vi "main.vi"(11 "librarian_sm.lvclass":refnum<class "librarian.lvclass">) -> ()   [LabVIEW 2020, in "librarian.lvclass"]
uses:
  librarian.lvclass
  typedefs/library--map.ctl
  typedefs/lib_map_value--cluster.ctl
  typedefs/book_state--enum.ctl
  shared/message--cluster.ctl
  shared/request--enum.ctl
  librarian.lvclass/librarian.ctl
  shared/_JKI_lib_State_Machine.llb/Select State(s)_err__jki_lib_state_machine.vi
panel:
  out "error out":errorcluster[](array[cluster])
  out "log":string
  in  "Exit":bool
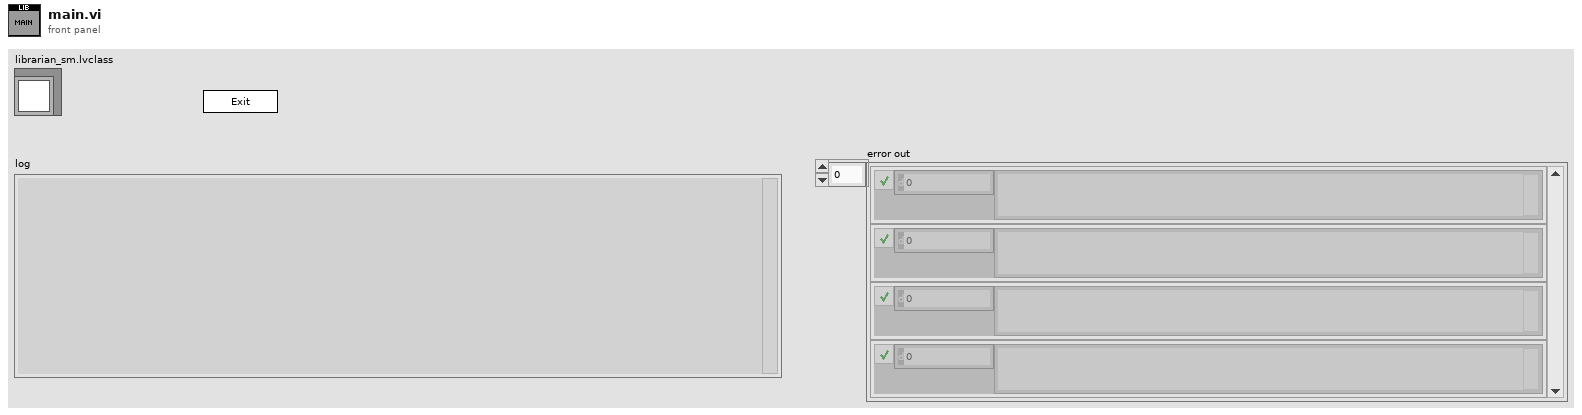
[diagram p1: front panel]
types:
  T1 = enum32{"Invalid", "Standard", "Closed", "Hidden", "Minimized", "Maximized"}
  T2 = enum32{"invalid app kind", "Development System", "Run Time System", "Student Edition", "Embedded LabVIEW", "Evaluation", "Custom"}
  T3 = typedef "librarian.lvclass/book_state--enum.ctl" = enum16{"CHECKEDIN", "CHECKEDOUT", "DAMAGED"}
  T4 = typedef "message--cluster.ctl" = cluster{"header":string, "cmd":T5, "title":string, "book":string}
  T5 = typedef "request--enum.ctl" = enum16{"CHECKIN", "CHECKOUT"}
  T6 = typedef "librarian.lvclass/lib_map_value--cluster.ctl" = cluster{"book state":T3, "text":string, "hash":string}
  T7 = typedef "librarian.lvclass/library--map.ctl" = map{string, T6}
  T8 = cluster{"Core":cluster{"Current VI Reference":refnum<vi>, "Close Panel on Exit?":bool}, "librarian_sm.lvclass":refnum<class "librarian.lvclass">, "TO":i32, "library map":T7, "listener ref":refnum<k5>, "client ref":refnum<k5>, "message":T4, "client map":map{string, cluster{"banned":bool, "title":string}}, "start time":u32}
  T9 = map{string, cluster{"banned":bool, "title":string}}
  T10 = cluster{"Current VI Reference":refnum<vi>, "Close Panel on Exit?":bool}
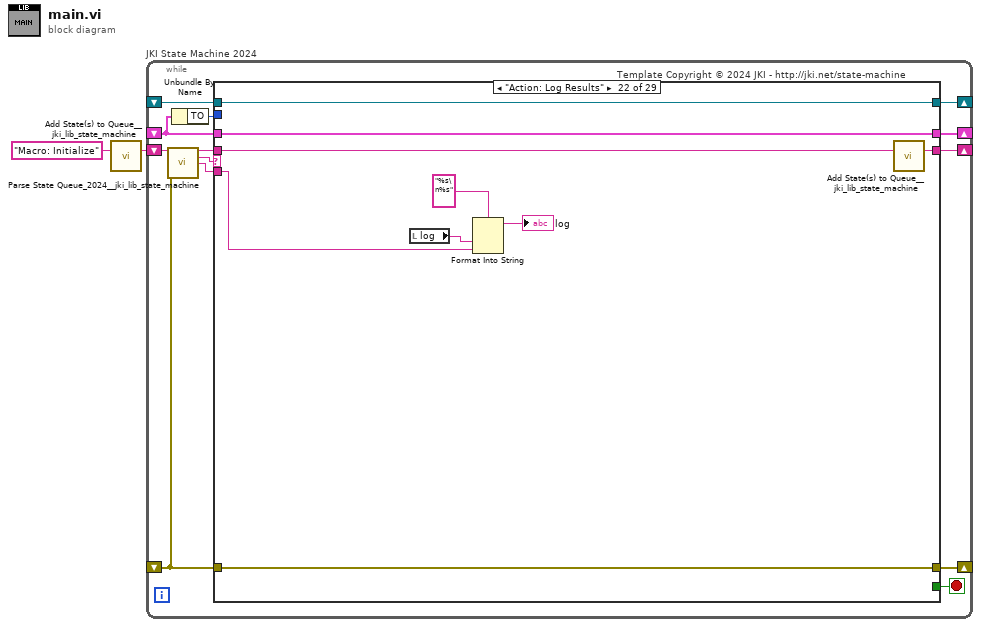
[diagram p0: block diagram]
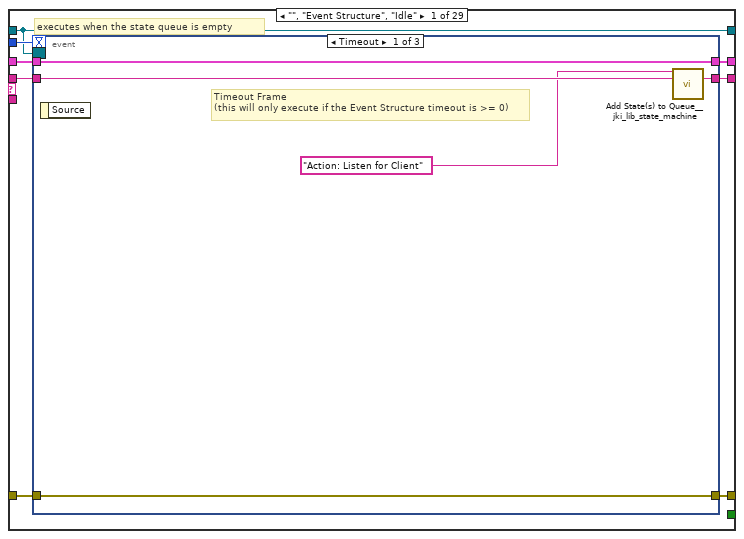
[diagram p2: hidden frame]
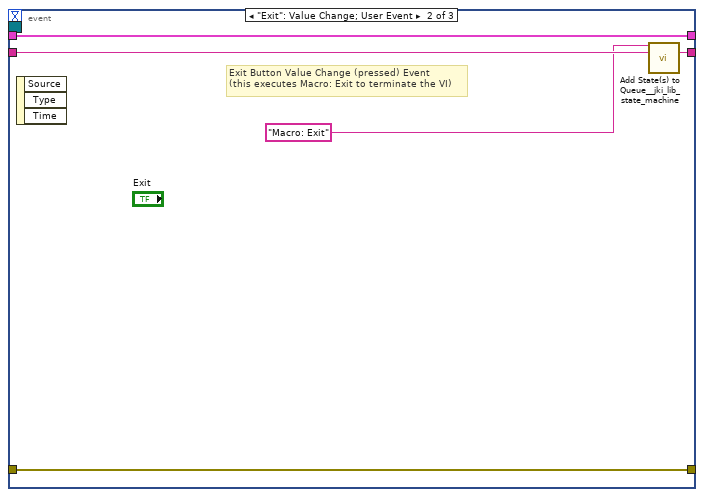
[diagram p3: hidden frame]
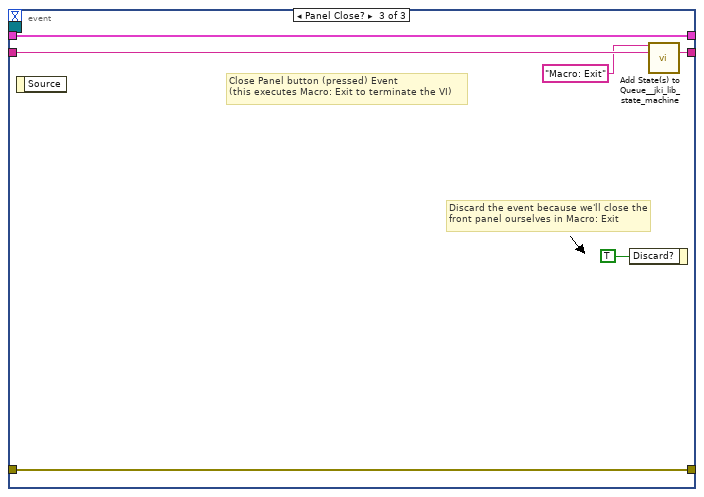
[diagram p4: hidden frame]
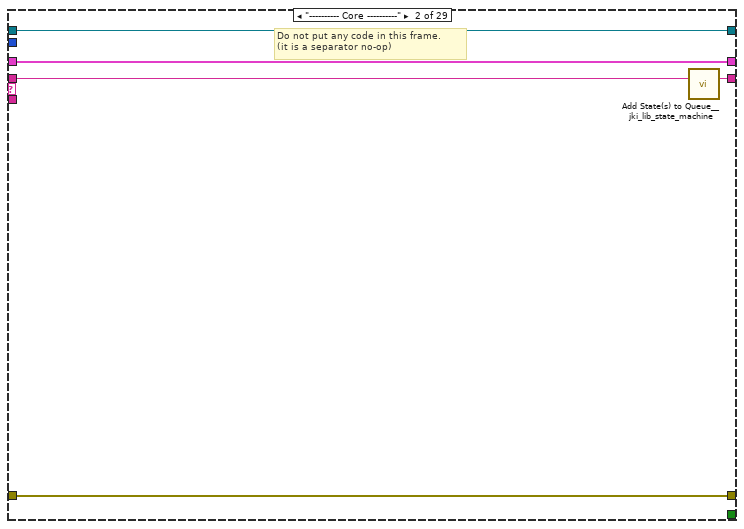
[diagram p5: hidden frame]
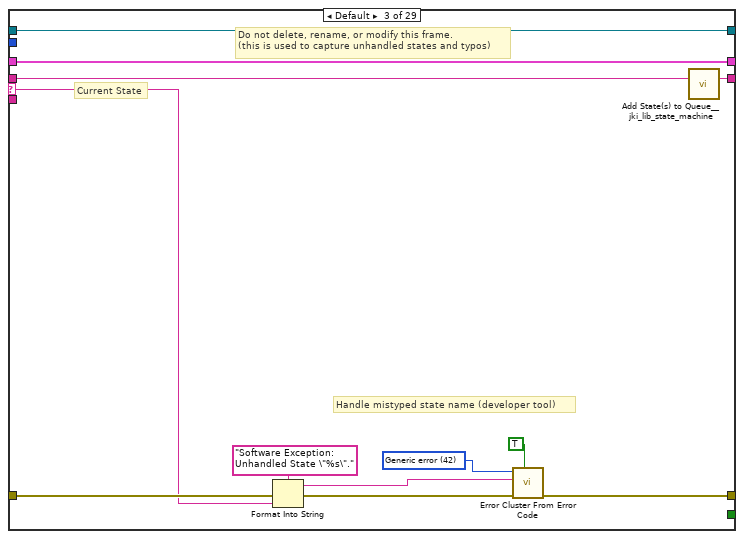
[diagram p6: hidden frame]
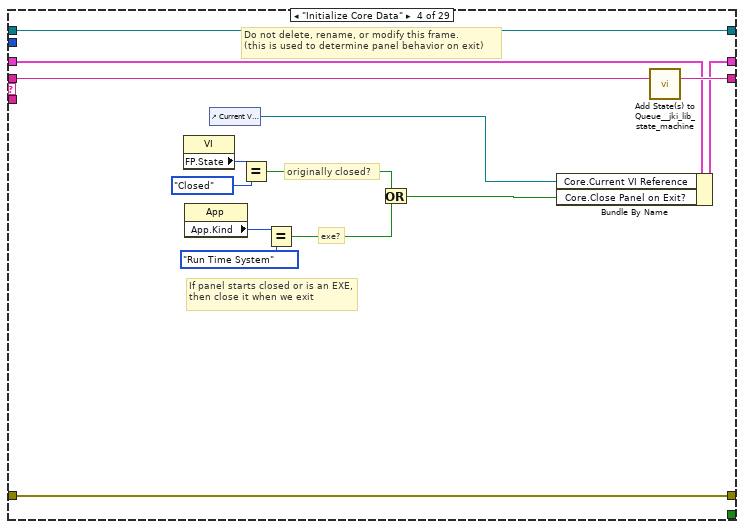
[diagram p7: hidden frame]
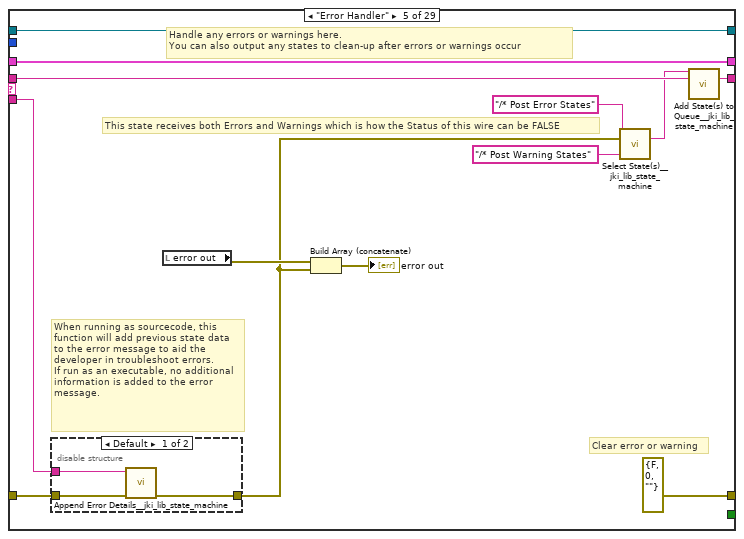
[diagram p8: hidden frame]
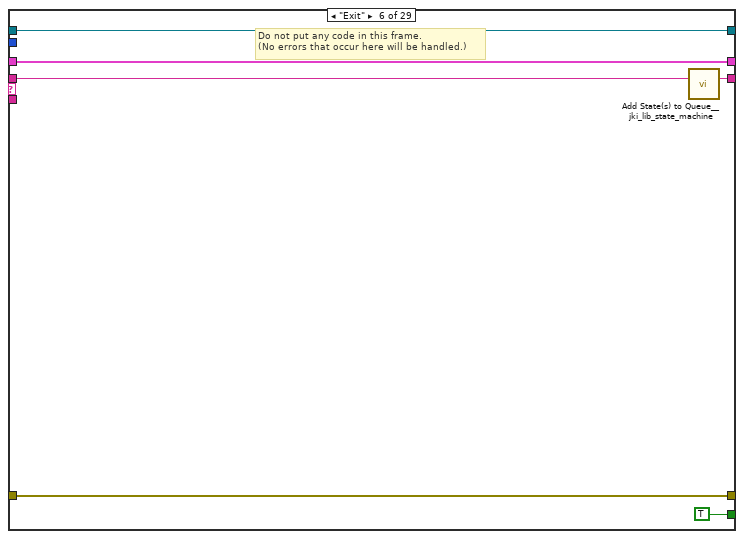
[diagram p10: hidden frame]
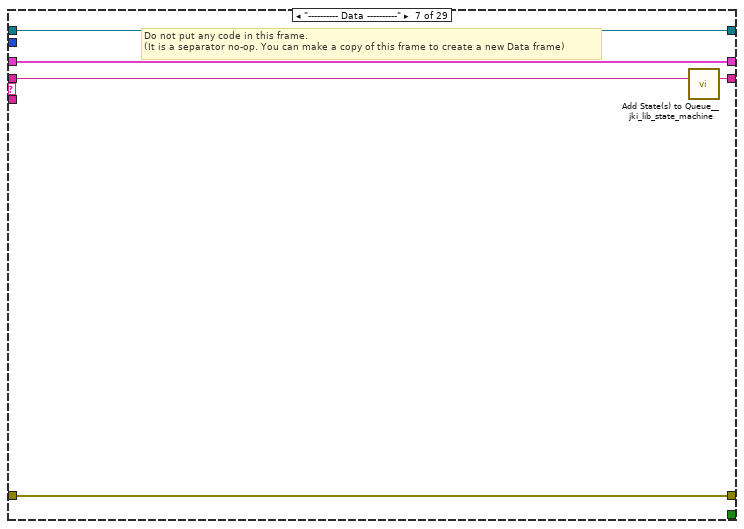
[diagram p11: hidden frame]
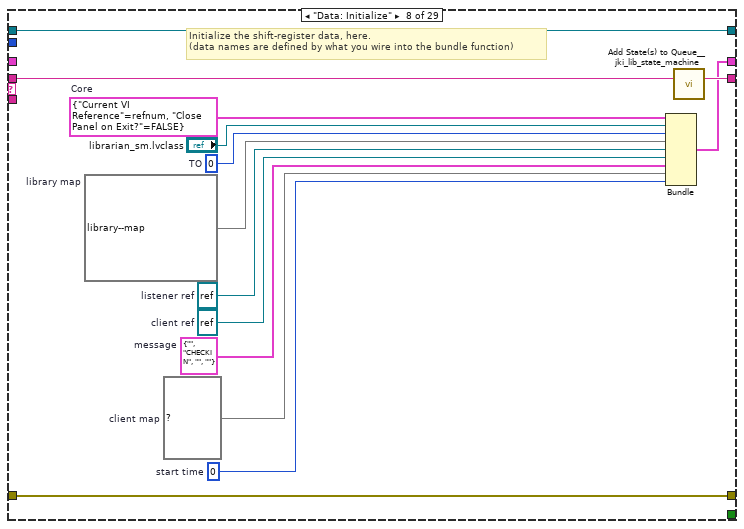
[diagram p12: hidden frame]
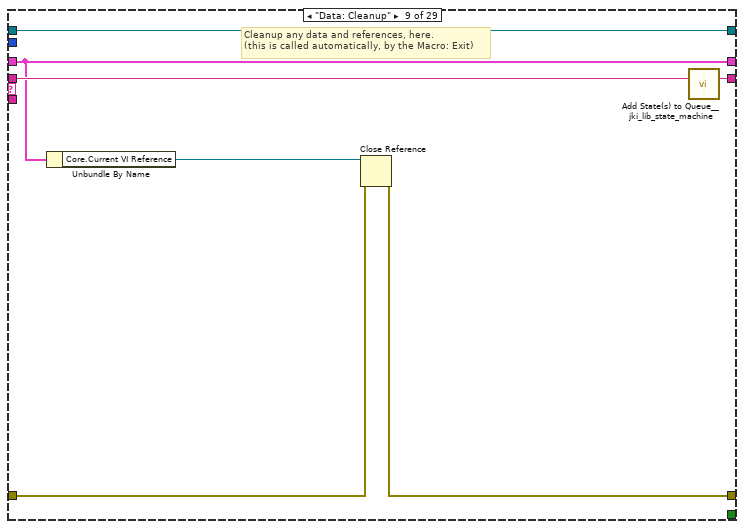
[diagram p13: hidden frame]
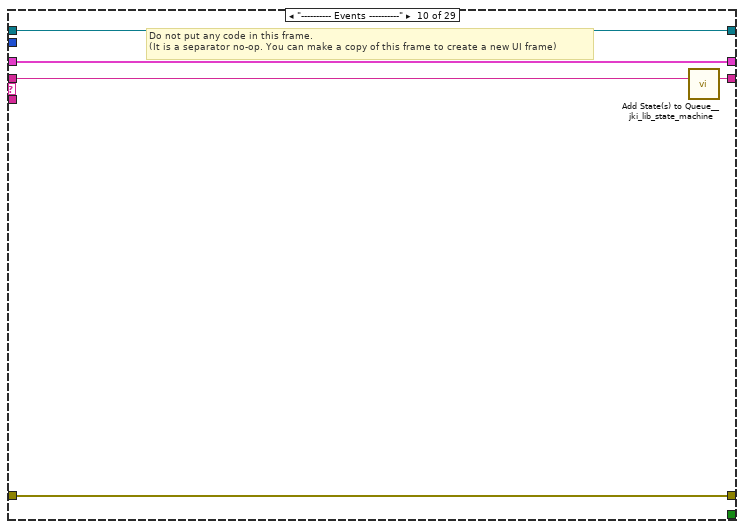
[diagram p14: hidden frame]
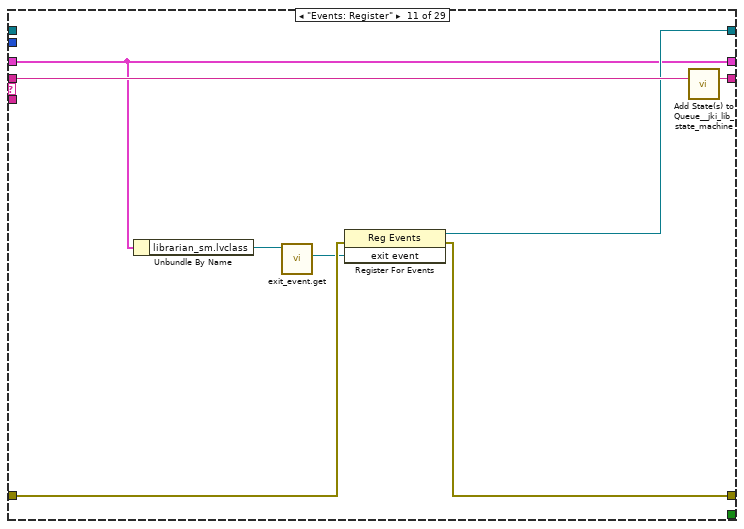
[diagram p15: hidden frame]
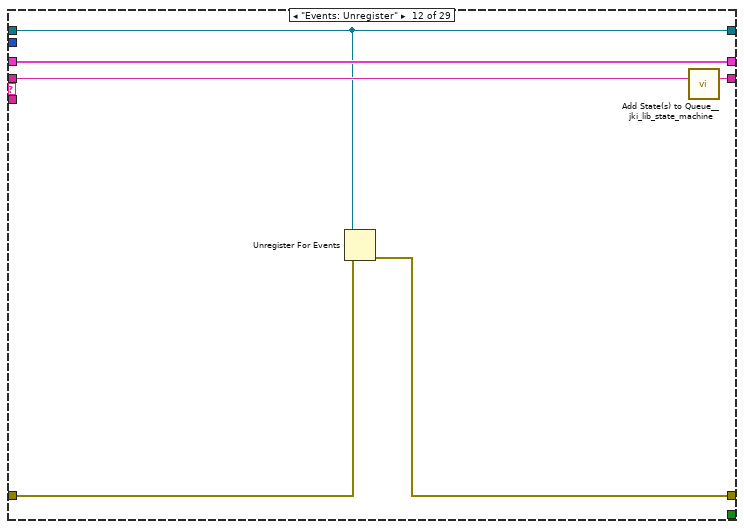
[diagram p16: hidden frame]
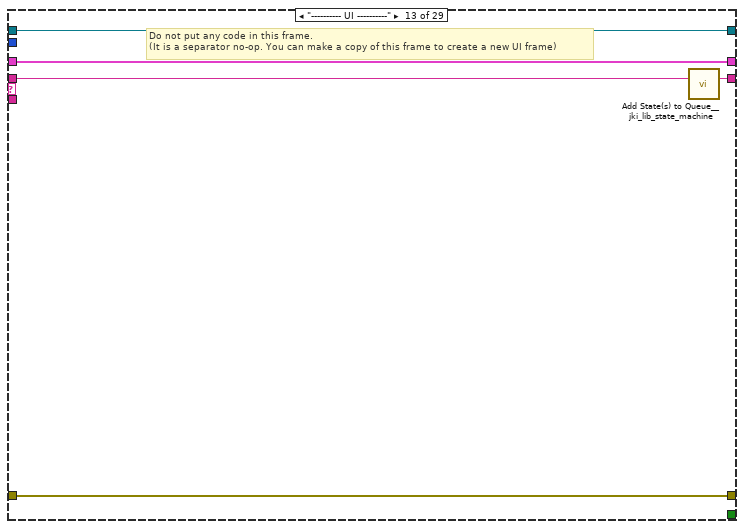
[diagram p17: hidden frame]
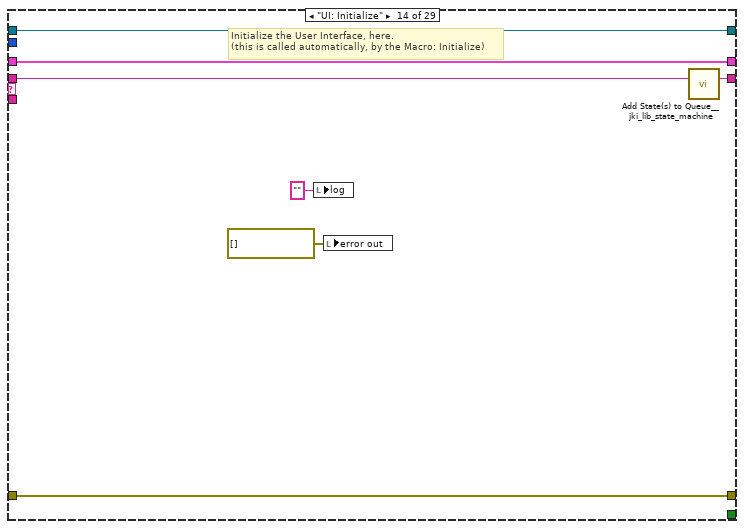
[diagram p18: hidden frame]
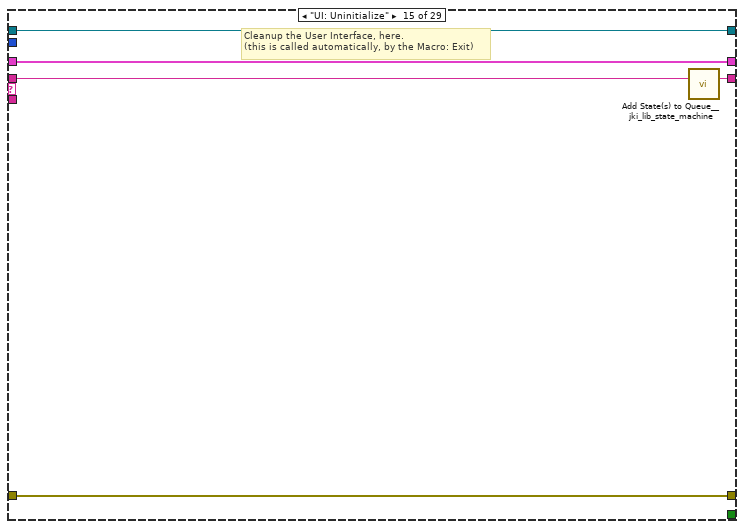
[diagram p19: hidden frame]
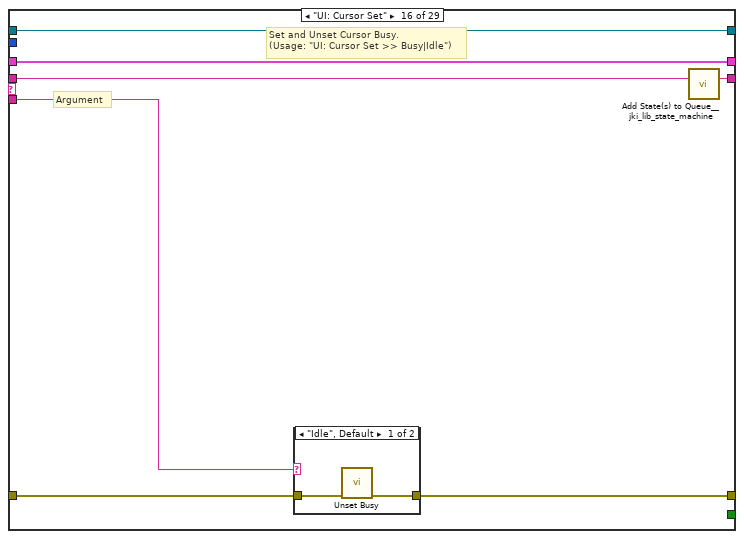
[diagram p20: hidden frame]
diagram:
  n1 = call "Add State(s) to Queue__jki_lib_state_machine.vi"("State(s) in (\"\")"="Macro: Initialize") -> ("States Out"=w2:string)  [unwired: 14 in]
  n2 = while "JKI State Machine 2024" {
    shift-right: [w8] -> _
    shift-left: _ -> [w4]
    shift-right: [w11] -> _
    shift-left: _ -> [w7]
    shift-right: [w10] -> _
    shift-left: w2 -> [w12]
    shift-right: [w6] -> _
    shift-left: _ -> [w5]
    stop <- w9 stop-if-true
    # "Template Copyright © 2024 JKI - http://jki.net/state-machine"
    n3 = call "Parse State Queue_2024__jki_lib_state_machine.vi"("State Queue"=w12, "Error In (no error)"=w7) -> ("Remaining States"=w14:string, "Current State"=w15:string, "Arguments"=w13:string)  [unwired: 11 in]
    n4 = Unbundle By Name(w4) -> ("TO"=w3:i32)
    n5 = case shown="\"Action: Log Results\"" w15 {
      selector: w15 -> [_ _ w46 _ _ _ _ _ _ _ _ _ _ _ _ _ _ _ _ _ _ _ _ _ _ _ _ _ _]
      tunnel: w14 -> [w23 w44 w50 w70 w83 w93 w98 w112 w119 w124 w132 w138 w143 w150 w155 w162 w174 w244 w250 w260 w265 w274 w295 w316 w363 w381 w406 w422 w434]
      tunnel: w13 -> [_ _ _ _ w78 _ _ _ _ _ _ _ _ _ _ w157 w168 _ _ _ _ w267 w283 _ _ _ _ _ _]
      tunnel: w4 -> [w21 w41 w48 w63 w80 w91 w95 _ w114 w121 w127 w136 w140 w148 w153 w160 w170 w241 w247 w258 w262 w271 w289 w307 w347 w370 w398 w419 w431]
      tunnel: [w20 w42 w52 w67 errorcluster {"status"=FALSE, "code"=0, "source"=""} ("error out") w90 w96 w109 w115 w122 w128 w133 w141 w147 w152 w158 w171 w242 w248 w255 w263 w272 w286 w314 w349 w367 w400 w416 w423] -> w11
      tunnel: w7 -> [w17 w42 w51 w67 w79 w90 w96 w109 w116 w122 w129 w134 w141 w147 w152 w159 w172 w242 w248 w255 w263 w272 w281 w314 w353 w375 w402 w417 w430]
      tunnel: [w22 w43 w49 w69 w82 w92 w97 w111 w118 w123 w131 w137 w142 w149 w154 w161 w173 w243 w249 w259 w264 w273 w294 w315 w362 w380 w405 w421 w433] -> w10
      tunnel: [_ _ _ _ _ TRUE _ _ _ _ _ _ _ _ _ _ _ _ _ _ _ _ _ _ _ _ _ _ _] -> w9
      tunnel: [w19 w41 w48 w68 w80 w91 w95 w110 w114 w121 w127 w136 w140 w148 w153 w160 w170 w241 w247 w258 w262 w271 w287 w305 w345 w369 w397 w419 w426] -> w8
      tunnel: w3 -> [w18 _ _ _ _ _ _ _ _ _ _ _ _ _ _ _ _ _ _ _ _ _ _ _ _ _ _ _ _]
      tunnel: [w16 w40 w45 w57 w74 w88 w94 w107 w113 w120 w130 w135 w139 w146 w151 w156 w167 w240 w245 w251 w261 w270 w293 w313 w361 w379 w404 w420 w432] -> w6
      tunnel: w5 -> [w16 w40 w45 w57 w74 w88 w94 w107 w113 w120 _ w135 w139 w146 w151 w156 w167 w240 w245 w251 w261 w270 w293 w313 w361 w379 w404 w420 w432]
      frame "", "Event Structure", "Idle" {
        # "executes when the state queue is empty"
        n6 = event shown="[0] Timeout" {
          selector: w16 -> [_ _ _]
          dyn-events: _ -> [_ _ _]
          timeout: w18 -> [_ _ _]
          tunnel: w23 -> [w28 w33 w39]
          tunnel: [w27 w32 w38] -> w22
          tunnel: w21 -> [w25 w30 w36]
          tunnel: [w26 w31 w37] -> w20
          tunnel: w17 -> [w26 w31 w37]
          tunnel: [w25 w30 w36] -> w19
          event Timeout {
            # "Timeout Frame\n(this will only execute if the Event Structure timeout is >= 0)"
            n7 = event-data() -> ()  [unwired: 1 in, 1 out]
            n8 = call "Add State(s) to Queue__jki_lib_state_machine.vi"("State(s) in Front (\"\")"="Action: Listen for Client" ("State"), "State(s) in (\"\")"=w28) -> ("States Out"=w27:string)  [unwired: 13 in]
          }
          event "Exit": Value Change; User Event {
            # "Exit Button Value Change (pressed) Event\n(this executes Macro: Exit to terminate the VI)"
            n9 = event-data() -> ()  [unwired: 1 in, 3 out]
            n10 = call "Add State(s) to Queue__jki_lib_state_machine.vi"("State(s) in Front (\"\")"="Macro: Exit", "State(s) in (\"\")"=w33) -> ("States Out"=w32:string)  [unwired: 13 in]
          }
          event Panel Close? {
            # "Discard the event because we'll close the front panel ourselves in Macro: Exit"
            # "Close Panel button (pressed) Event\n(this executes Macro: Exit to terminate the VI)"
            n11 = event-data() -> ()  [unwired: 1 in, 1 out]
            n12 = event-data("Discard?"=TRUE) -> ()  [unwired: 1 in, 1 out]
            n13 = call "Add State(s) to Queue__jki_lib_state_machine.vi"("State(s) in Front (\"\")"="Macro: Exit", "State(s) in (\"\")"=w39) -> ("States Out"=w38:string)  [unwired: 13 in]
          }
        }
      }
      frame "---------- Core ----------" {
        # "Do not put any code in this frame.\n(it is a separator no-op)"
        n14 = call "Add State(s) to Queue__jki_lib_state_machine.vi"("State(s) in (\"\")"=w44) -> ("States Out"=w43:string)  [unwired: 14 in]
      }
      frame Default {
        w55 = 42 items=["No error", "Argument error", "Memory is full", "Out of zone", "End of file", "File already open", "Generic file I/O error", "File not found", "File permission error", "Disk is full", "Duplicate path", "Too many files open", "System feature not enabled", "Resource file not found", "Cannot add resource", "Resource not found", "Image not found", "Image memory error", "Pen does not exist", "Config type invalid", "Config token not found", "Config parse error", "Config memory error", "Bad external code format", "Bad external code offset", "External code not present", "Null window", "Destroy window error", "Null menu", "Print aborted", "Bad print record", "Print driver error", "Windows error during printing", "Memory error during printing", "Print dialog error", "Generic print error", "Invalid device refnum", "Device not found", "Device parameter error", "Device unit error", "Cannot open device", "Device call aborted", "Generic error", "Cancelled by user", "Object ID too low", "Object ID too high", "Object not in heap", "Unknown heap", "Unknown object (invalid DefProc)", "Unknown object (DefProc not in table)", "Message out of range", "Invalid (null) method", "Unknown message", "Manager call not supported", "Bad address", "Network operation in progress", "Network operation timed out", "Connection is busy", "Network attribute not supported", "Network error", "Address in use", "System out of memory", "Connection aborted", "Connection refused", "Not connected", "Already connected", "Connection closed", "Initialization error (interapplication manager)", "Bad occurrence", "Wait on unbound occurrence handler", "Occurrence queue overflow", "Datalog type conflict", "Unused", "Unrecognized type (interapplication manager)", "Memory corrupt", "Failed to make temporary DLL", "Old CIN version", "Drag socket not found", "Failed to load drop-object", "Failed to register OLE object", "Failed to release OLE object", "Format specifier type mismatch", "Unknown format specifier", "Too few format specifiers", "Too many format specifiers", "Scan failed", "Newer CIN version", "Error converting to variant", "Runtime menu error", "Password tampered", "Variant attribute not found", "Incompatible variant data type", "Event data is not available", "Event Store is not present", "Occurrence is not found", "Event Queue is not created", "Event info is not available", "Refnum passed is NULL", "Error retrieving Class GUID", "Error retrieving CoClass GUID", "Error retrieving TypeLib GUID.", "Bad built application magic bytes.", "Specific driver is different from the specific driver associated with the Logical Name.", "There is no session opened to the class driver.", "Max Error", "MAX - Error with config objects", "MAX - Error loading configuration", "MAX - Group not supported"]
        # "Current State"
        # "Do not delete, rename, or modify this frame.\n(this is used to capture unhandled states and typos)"
        # "Handle mistyped state name (developer tool)"
        n15 = Format Into String(format string="Software Exception: Unhandled State \"%s\"." ("message"), error in=w51, w46) -> (resulting string=w54:string, error out=w53:errorcluster)  [unwired: 1 in]
        n16 = call <vilib>:"Error Cluster From Error Code.vi"("show call chain? (False)"=TRUE, "error in (no error)"=w53, "error message (\"\")"=w54, "error code (0)"=w55) -> ("error out"=w52:errorcluster)  [unwired: 5 in]
        n17 = call "Add State(s) to Queue__jki_lib_state_machine.vi"("State(s) in (\"\")"=w50) -> ("States Out"=w49:string)  [unwired: 14 in]
      }
      frame "Initialize Core Data" {
        # "Do not delete, rename, or modify this frame.\n(this is used to determine panel behavior on exit)"
        # "originally closed?"
        # "exe?"
        # "If panel starts closed or is an EXE, then close it when we exit"
        n18 = property class="VI"() -> ("FP.State"=w60:T1)  [unwired: 2 in, 2 out]
        n19 = property class="App"() -> ("App.Kind"=w66:T2)  [unwired: 2 in, 2 out]
        n20 = control-ref of="Current VI Reference"() -> (w61:refnum<vi>)
        n21 = Equal?(x=w60, y=T1."Closed" ("Front Panel Window:State")) -> (x = y?=w58:bool)
        n22 = Equal?(x=w66, y=T2."Run Time System" ("Application:Kind")) -> (x = y?=w64:bool)
        n23 = Or(x=w58, y=w64) -> (x .or. y?=w62:bool)
        n24 = Bundle By Name(cluster=w63, "Core.Current VI Reference"=w61, "Core.Close Panel on Exit?"=w62) -> (w68:T8)
        n25 = call "Add State(s) to Queue__jki_lib_state_machine.vi"("State(s) in (\"\")"=w70) -> ("States Out"=w69:string)  [unwired: 14 in]
      }
      frame "Error Handler" {
        # "When running as sourcecode, this function will add previous state data to the error message to aid the developer in troubleshoot errors.\nIf run as an executable, no additional information is added to the error message."
        # "This state receives both Errors and Warnings which is how the Status of this wire can be FALSE"
        # "Handle any errors or warnings here.\nYou can also output any states to clean-up after errors or warnings occur"
        # "Clear error or warning"
        n26 = disable-structure shown="Default" {
          disable-tunnel: w79 -> [w86 w87]
          disable-tunnel: w78 -> [w85 _]
          disable-tunnel: [w84 w87] -> w72
          frame condition #0 (active) {
            n27 = call "Append Error Details__jki_lib_state_machine.vi"("error in (no error)"=w86, "Previous State and Argument(s)"=w85) -> ("error out"=w84:errorcluster)  [unwired: 9 in]
          }
          frame condition #1 {
          }
        }
        n28 = local read "error out"() -> (w73:errorcluster[])
        n29 = Build Array (concatenate)(w73, w72) -> (→"error out":errorcluster[])
        n30 = call-poly "Select State(s)__jki_lib_state_machine.vi"("State(s) if True (\"\")"="/* Post Error States", "Select"=w72, "State(s) if False (\"\")"="/* Post Warning States") -> ("States Out"=w76:string)  [unwired: 12 in]
        n31 = call "Add State(s) to Queue__jki_lib_state_machine.vi"("State(s) in Front (\"\")"=w76, "State(s) in (\"\")"=w83) -> ("States Out"=w82:string)  [unwired: 13 in]
      }
      frame "Exit" {
        # "Do not put any code in this frame.\n(No errors that occur here will be handled.)"
        n32 = call "Add State(s) to Queue__jki_lib_state_machine.vi"("State(s) in (\"\")"=w93) -> ("States Out"=w92:string)  [unwired: 14 in]
      }
      frame "---------- Data ----------" {
        # "Do not put any code in this frame.\n(It is a separator no-op. You can make a copy of this frame to create a new Data frame)"
        n33 = call "Add State(s) to Queue__jki_lib_state_machine.vi"("State(s) in (\"\")"=w98) -> ("States Out"=w97:string)  [unwired: 14 in]
      }
      frame "Data: Initialize" {
        w99 = u32 0  # start time
        w100 = T9 {}  # client map
        w101 = T4 {"header"="", "cmd"=enum."CHECKIN", "title"="", "book"=""}  # message
        w102 = refnum<k5> refnum  # client ref
        w103 = refnum<k5> refnum  # listener ref
        w104 = T7 {}  # library map
        w105 = 0  # TO
        w108 = T10 {"Current VI Reference"=refnum, "Close Panel on Exit?"=FALSE}  # Core
        # "Initialize the shift-register data, here.\n(data names are defined by what you wire into the bundle function)"
        n34 = Bundle("Core"=w108, "librarian_sm.lvclass"="librarian_sm.lvclass", "TO"=w105, "library map"=w104, "listener ref"=w103, "client ref"=w102, "message"=w101, "client map"=w100, "start time"=w99) -> (w110:T8)  [unwired: 1 in]
        n35 = call "Add State(s) to Queue__jki_lib_state_machine.vi"("State(s) in (\"\")"=w112) -> ("States Out"=w111:string)  [unwired: 14 in]
      }
      frame "Data: Cleanup" {
        # "Cleanup any data and references, here.\n(this is called automatically, by the Macro: Exit)"
        n36 = Unbundle By Name(w114) -> ("Core.Current VI Reference"=w117:refnum<vi>)
        n37 = Close Reference(reference=w117, error in (no error)=w116) -> (error out=w115:errorcluster)
        n38 = call "Add State(s) to Queue__jki_lib_state_machine.vi"("State(s) in (\"\")"=w119) -> ("States Out"=w118:string)  [unwired: 14 in]
      }
      frame "---------- Events ----------" {
        # "Do not put any code in this frame.\n(It is a separator no-op. You can make a copy of this frame to create a new UI frame)"
        n39 = call "Add State(s) to Queue__jki_lib_state_machine.vi"("State(s) in (\"\")"=w124) -> ("States Out"=w123:string)  [unwired: 14 in]
      }
      frame "Events: Register" {
        n40 = Unbundle By Name(w127) -> ("librarian_sm.lvclass"=w126:refnum<class "librarian.lvclass">)
        n41 = call "exit_event.get.vi"("librarian_sm in"=w126) -> ("exit event"=w125:refnum<user-event>)  [unwired: 9 in, 1 out]
        n42 = register-events(error in=w129, w125) -> (reference out=w130:refnum<event-registration>, error out=w128:errorcluster)  [unwired: 1 in]
        n43 = call "Add State(s) to Queue__jki_lib_state_machine.vi"("State(s) in (\"\")"=w132) -> ("States Out"=w131:string)  [unwired: 14 in]
      }
      frame "Events: Unregister" {
        n44 = Unregister For Events(event registration refnum=w135, error in=w134) -> (error out=w133:errorcluster)
        n45 = call "Add State(s) to Queue__jki_lib_state_machine.vi"("State(s) in (\"\")"=w138) -> ("States Out"=w137:string)  [unwired: 14 in]
      }
      frame "---------- UI ----------" {
        # "Do not put any code in this frame.\n(It is a separator no-op. You can make a copy of this frame to create a new UI frame)"
        n46 = call "Add State(s) to Queue__jki_lib_state_machine.vi"("State(s) in (\"\")"=w143) -> ("States Out"=w142:string)  [unwired: 14 in]
      }
      frame "UI: Initialize" {
        # "Initialize the User Interface, here.\n(this is called automatically, by the Macro: Initialize)"
        n47 = local write "log"("" ("log")) -> ()
        n48 = local write "error out"(errorcluster[] [] ("error out")) -> ()
        n49 = call "Add State(s) to Queue__jki_lib_state_machine.vi"("State(s) in (\"\")"=w150) -> ("States Out"=w149:string)  [unwired: 14 in]
      }
      frame "UI: Uninitialize" {
        # "Cleanup the User Interface, here.\n(this is called automatically, by the Macro: Exit)"
        n50 = call "Add State(s) to Queue__jki_lib_state_machine.vi"("State(s) in (\"\")"=w155) -> ("States Out"=w154:string)  [unwired: 14 in]
      }
      frame "UI: Cursor Set" {
        # "Argument"
        # "Set and Unset Cursor Busy.\n(Usage: \"UI: Cursor Set >> Busy|Idle\")"
        n51 = case shown="\"Idle\", Default" w157 {
          tunnel: w159 -> [w164 w166]
          tunnel: [w163 w165] -> w158
          frame "Idle", Default {
            n52 = call <vilib>:"Unset Busy.vi"("error in (no error)"=w164) -> ("error out"=w163:errorcluster)  [unwired: 10 in]
          }
          frame "Busy" {
            n53 = call <vilib>:"Set Busy.vi"("error in (no error)"=w166) -> ("error out"=w165:errorcluster)  [unwired: 9 in, 1 out]
          }
        }
        n54 = call "Add State(s) to Queue__jki_lib_state_machine.vi"("State(s) in (\"\")"=w162) -> ("States Out"=w161:string)  [unwired: 14 in]
      }
      frame "UI: Front Panel State" {
        # "Argument"
        # "Set Front Panel Open or Closed\n(Usage: \"UI: Front Panel State >> Open|Close\")"
        n55 = Unbundle By Name(w170) -> ("Core.Current VI Reference"=w169:refnum<vi>)
        n56 = case shown="\"Minimize\", \"Minimized\"" w168 {
          tunnel: w172 -> [w180 w195 w206 w219 w232]
          tunnel: [w182 w196 w208 w221 w234] -> w171
          tunnel: w169 -> [w181 w193 w207 w220 w233]
          frame "Open", "Standard", Default {
            w175 = T1."Standard" ("State")
            n57 = property class="VI"(reference=w181, error in=w180) -> (reference out=w178:refnum<vi>, error out=w179:errorcluster, "FP.State"=w177:T1)
            n58 = Not Equal?(x=w177, y=w175) -> (x != y?=w176:bool)
            n59 = case shown="True" w176 {
              tunnel: [w186 w188] -> w182
              tunnel: w179 -> [w185 w188]
              tunnel: w178 -> [w184 _]
              tunnel: w175 -> [w183 _]
              frame True {
                n60 = invoke class="VI" method="FP.Open"(reference=w184, error in=w185, "Activate"=TRUE, "State"=w183) -> (error out=w186:errorcluster)  [unwired: 1 in, 4 out]
              }
              frame False {
              }
            }
          }
          frame "Close", "Closed" {
            n61 = property class="VI"(reference=w193, error in=w195) -> (reference out=w192:refnum<vi>, error out=w194:errorcluster, "FP.State"=w190:T1)
            n62 = Not Equal?(x=w190, y=T1."Closed" ("Front Panel Window:State")) -> (x != y?=w189:bool)
            n63 = case shown="True" w189 {
              tunnel: [w197 w200] -> w196
              tunnel: w194 -> [w197 w199]
              tunnel: w192 -> [_ w198]
              frame False {
              }
              frame True {
                n64 = invoke class="VI" method="FP.Close"(reference=w198, error in=w199) -> (error out=w200:errorcluster)  [unwired: 1 in, 2 out]
              }
            }
          }
          frame "Hidden", "Hide" {
            w201 = T1."Hidden" ("State")
            n65 = property class="VI"(reference=w207, error in=w206) -> (reference out=w204:refnum<vi>, error out=w205:errorcluster, "FP.State"=w203:T1)
            n66 = Not Equal?(x=w203, y=w201) -> (x != y?=w202:bool)
            n67 = case shown="True" w202 {
              tunnel: [w212 w213] -> w208
              tunnel: w205 -> [w211 w213]
              tunnel: w204 -> [w210 _]
              tunnel: w201 -> [w209 _]
              frame True {
                n68 = invoke class="VI" method="FP.Open"(reference=w210, error in=w211, "State"=w209) -> (error out=w212:errorcluster)  [unwired: 2 in, 4 out]
              }
              frame False {
              }
            }
          }
          frame "Minimize", "Minimized" {
            w214 = T1."Minimized" ("State")
            n69 = property class="VI"(reference=w220, error in=w219) -> (reference out=w217:refnum<vi>, error out=w218:errorcluster, "FP.State"=w216:T1)
            n70 = Not Equal?(x=w216, y=w214) -> (x != y?=w215:bool)
            n71 = case shown="True" w215 {
              tunnel: [w225 w226] -> w221
              tunnel: w218 -> [w224 w226]
              tunnel: w217 -> [w223 _]
              tunnel: w214 -> [w222 _]
              frame True {
                n72 = invoke class="VI" method="FP.Open"(reference=w223, error in=w224, "State"=w222) -> (error out=w225:errorcluster)  [unwired: 2 in, 4 out]
              }
              frame False {
              }
            }
          }
          frame "Maximize", "Maximized" {
            w227 = T1."Maximized" ("State")
            n73 = property class="VI"(reference=w233, error in=w232) -> (reference out=w230:refnum<vi>, error out=w231:errorcluster, "FP.State"=w229:T1)
            n74 = Not Equal?(x=w229, y=w227) -> (x != y?=w228:bool)
            n75 = case shown="True" w228 {
              tunnel: [w238 w239] -> w234
              tunnel: w231 -> [w237 w239]
              tunnel: w230 -> [w236 _]
              tunnel: w227 -> [w235 _]
              frame True {
                n76 = invoke class="VI" method="FP.Open"(reference=w236, error in=w237, "State"=w235) -> (error out=w238:errorcluster)  [unwired: 2 in, 4 out]
              }
              frame False {
              }
            }
          }
        }
        n77 = call "Add State(s) to Queue__jki_lib_state_machine.vi"("State(s) in (\"\")"=w174) -> ("States Out"=w173:string)  [unwired: 14 in]
      }
      frame "---------- Macro ----------" {
        # "Do not put any code in this frame.\n(It is a separator no-op. You can make a copy of this frame to create a new Macro frame)"
        n78 = call "Add State(s) to Queue__jki_lib_state_machine.vi"("State(s) in (\"\")"=w244) -> ("States Out"=w243:string)  [unwired: 14 in]
      }
      frame "Macro: Initialize" {
        # "Initialization Macro\n(This is called once, when the VI starts)"
        n79 = call "Add State(s) to Queue__jki_lib_state_machine.vi"("State(s) in Front (\"\")"="Data: Initialize\nInitialize Core Data\nEvents: Register\nUI: Initialize\nUI: Front Panel State >> Open\nAction: Open Listener\nAction: Load Library", "State(s) in (\"\")"=w250) -> ("States Out"=w249:string)  [unwired: 13 in]
      }
      frame "Macro: Exit" {
        # "Exit Macro\n(This is called once, when the VI exits)"
        n80 = Unbundle By Name(w258) -> ("Core.Close Panel on Exit?"=w253:bool)
        n81 = call "Conditional State String__jki_lib_state_machine.vi"("Do State(s)?"=w253, "State"="UI: Front Panel State >> Close") -> ("State Out"=w252:string)  [unwired: 7 in]
        n82 = call "Add State(s) to Queue__jki_lib_state_machine.vi"("State(s) in (\"\")"=w252, "State(s) at Back (\"\")"="Action: Close TCP Port\nUI: Uninitialize\nData: Cleanup\nEvents: Unregister\nExit") -> ("States Out"=w256:string)  [unwired: 13 in]
        n83 = call "Add State(s) to Queue__jki_lib_state_machine.vi"("State(s) in Front (\"\")"=w256, "State(s) in (\"\")"=w260) -> ("States Out"=w259:string)  [unwired: 13 in]
      }
      frame "---------- Action ----------" {
        n84 = call "Add State(s) to Queue__jki_lib_state_machine.vi"("State(s) in (\"\")"=w265) -> ("States Out"=w264:string)  [unwired: 14 in]
      }
      frame "Action: Log Results" {
        n85 = local read "log"() -> (w268:string)
        n86 = Format Into String(format string="%s\n%s", w268, w267) -> (resulting string=→"log":string)  [unwired: 2 in, 1 out]
        n87 = call "Add State(s) to Queue__jki_lib_state_machine.vi"("State(s) in (\"\")"=w274) -> ("States Out"=w273:string)  [unwired: 14 in]
      }
      frame "Action: Checkout book" {
        n88 = Unbundle By Name(w289) -> ("library map"=w291:T7, "start time"=w280:u32, "client ref"=w279:refnum<k5>, "message.header"=w278:string)
        n89 = Look In Map(map=w291, key=w283) -> (value=w290:T6)  [unwired: 1 in, 1 out]
        n90 = Unbundle By Name(w290) -> ("book state"=w292:T3)
        n91 = case shown="\"CHECKEDIN\"" w292 {
          tunnel: w291 -> [w300 w303]
          tunnel: w290 -> [w302 _]
          tunnel: w283 -> [w297 _]
          tunnel: [w298 w303] -> w288
          tunnel: [w296 _] -> w282
          frame "CHECKEDIN" {
            # "Book available. Checkout"
            n92 = Unbundle By Name(w302) -> ("text"=w296:string)
            n93 = Bundle By Name(cluster=w302, "book state"=book_state--enum."CHECKEDOUT") -> (w299:T6)
            n94 = Insert Into Map(map in=w300, key=w297, value=w299) -> (map out=w298:T7)  [unwired: 2 out]
          }
          frame "CHECKEDOUT", Default {
            # "Book is either checkout or damaged"
          }
        }
        n95 = call "send_book.vi"("client id"=w278, "start time"=w280, "error in (no error)"=w281, "book"=w282, "title"=w283, "client tcp ref"=w279) -> ("error out"=w284:errorcluster, "log string"=w276:string, "client tcp ref out"=w285:refnum<k5>)  [unwired: 3 in]
        n96 = TCP Close Connection(connection ID=w285, error in (no error)=w284) -> (error out=w286:errorcluster)  [unwired: 1 in, 1 out]
        n97 = Bundle By Name(cluster=w289, "library map"=w288) -> (w287:T8)
        n98 = Concatenate Strings("Action: Log Results >> ", w276) -> (w275:string)
        n99 = call "Add State(s) to Queue__jki_lib_state_machine.vi"("State(s) in Front (\"\")"=w275, "State(s) in (\"\")"=w295) -> ("States Out"=w294:string)  [unwired: 13 in]
      }
      frame "Action: Process Checkout" {
        n100 = Unbundle By Name(w307) -> ("client map"=w309:T9, "message.header"=w310:string, "message.title"=w311:string)
        n101 = Look In Map(map=w309, key=w310) -> (key not found?=w312:bool, value=w304:cluster{"banned":bool, "title":string})  [unwired: 1 in]
        n102 = case shown="True" w312 {
          tunnel: w311 -> [w318 w342]
          tunnel: w310 -> [w317 w339]
          tunnel: w309 -> [w319 w340]
          tunnel: [w321 w341] -> w308
          tunnel: [w319 w337] -> w306
          tunnel: w304 -> [w323 _]
          frame False {
            # "Existing Client.  Check status and make sure nothing is already checked out"
            n103 = Unbundle By Name(w323) -> ("banned"=w322:bool, "title"=w320:string)
            n104 = case shown="False" w322 {
              tunnel: [w325 "Action: Reply Banned"] -> w321
              tunnel: w320 -> [w328 _]
              tunnel: w318 -> [w326 _]
              tunnel: w317 -> [w324 _]
              frame False {
                # "Check for book checked out"
                n105 = Empty String/Path?(string/path=w328) -> (empty?=w327:bool)
                n106 = case shown="False" w327 {
                  tunnel: w326 -> [_ w334]
                  tunnel: [w330 w333] -> w325
                  tunnel: w324 -> [w331 _]
                  frame False {
                    # "Already checkedout"
                    n107 = Concatenate Strings("Action: Retrieve Book >> ", w331, "Action: Ban Client\nAction: Reply Banned") -> (w330:string)
                  }
                  frame True {
                    # "Good to checkout"
                    n108 = Concatenate Strings("Action: Checkout book >> ", w334) -> (w333:string)
                  }
                }
              }
              frame True {
                # "Client banned. Reply banned"
              }
            }
          }
          frame True {
            # "New client.  Add client and checkout title"
            n109 = Insert Into Map(map in=w340, key=w339, value=cluster{"banned":bool, "title":string} {"banned"=FALSE, "title"=""}) -> (map out=w337:T9)  [unwired: 2 out]
            n110 = Concatenate Strings("Action: Checkout book >> ", w342) -> (w341:string)
          }
        }
        n111 = Bundle By Name(cluster=w307, "client map"=w306) -> (w305:T8)
        n112 = call "Add State(s) to Queue__jki_lib_state_machine.vi"("State(s) in Front (\"\")"=w308, "State(s) in (\"\")"=w316) -> ("States Out"=w315:string)  [unwired: 13 in]
      }
      frame "Action: Get Client Request" {
        w355 = 1000  # timout
        w356 = 4  # I32
        n113 = Unbundle By Name(w347) -> ("client ref"=w354:refnum<k5>)
        n114 = TCP Read(connection ID=w354, bytes to read=w356, error in (no error)=w353, 9:w355) -> (connection ID out=w357:refnum<k5>, data out=w360:string, error out=w359:errorcluster)  [unwired: 1 out]
        n115 = Type Cast(type=w356, x=w360) -> (*(type *) &x=w358:i32)
        n116 = TCP Read(connection ID=w357, bytes to read=w358, error in (no error)=w359, 9:w355) -> (data out=w352:string, error out=w350:errorcluster)  [unwired: 2 out]
        n117 = Unflatten From String(type=T4 {"header"="", "cmd"=enum."CHECKIN", "title"="", "book"=""} ("request"), binary string=w352, error in (no error)=w350) -> (value=w346:T4, error out=w349:errorcluster)  [unwired: 2 in, 1 out]
        n118 = Unbundle By Name(w346) -> ("cmd"=w348:T5)
        n119 = Bundle By Name(cluster=w347, "message"=w346) -> (w345:T8)
        n120 = case shown="\"CHECKIN\"" w348 {
          tunnel: ["Action: Process Checkout" "Action: Process Checkout"] -> w344
          frame "CHECKIN" {
          }
          frame "CHECKOUT" {
          }
        }
        n121 = call "Add State(s) to Queue__jki_lib_state_machine.vi"("State(s) in Front (\"\")"=w344, "State(s) in (\"\")"=w363) -> ("States Out"=w362:string)  [unwired: 13 in]
      }
      frame "Action: Load Library" {
        w371 = T7 {}  # library map
        # "Load Library.\n(Read Library folder files and build Libray Map)"
        n122 = call <vilib>:"Application Directory.vi"() -> ("Application Directory"=w378:path)
        n123 = Build Path(base path=w378, name or relative path=path "Library") -> (appended path=w376:path)
        n124 = List Folder(path=w376, error in=w375) -> (path out=w372:path, filenames=w373:string[], error out=w374:errorcluster)  [unwired: 2 in, 1 out]
        n125 = for {
          shift-right: [w390] -> w367
          shift-left: w374 -> [w392]
          tunnel: w373 -> [w383] mode=indexing
          tunnel: w372 -> [w394]
          shift-right: [w382] -> w368
          shift-left: w371 -> [w385]
          n126 = Build Path(base path=w394, name or relative path=w383) -> (appended path=w393:path)
          n127 = Read from Text File(file (use dialog)=w393, error in=w392) -> (text=w387:string, error out=w391:errorcluster)  [unwired: 2 in, 2 out]
          n128 = call "SHA256_hash.vi"("error in (no error)"=w391, "text in"=w387) -> ("error out"=w390:errorcluster, "hash out"=w386:string)  [unwired: 8 in]
          n129 = Bundle By Name(cluster=T6 {"book state"=enum."CHECKEDIN", "text"="", "hash"=""} ("value"), "book state"=book_state--enum."CHECKEDIN", "text"=w387, "hash"=w386) -> (w384:T6)
          n130 = Insert Into Map(map in=w385, key=w383, value=w384) -> (map out=w382:T7)  [unwired: 2 out]
        }
        n131 = Tick Count (ms)() -> (millisecond timer value=w366:u32)
        n132 = Bundle By Name(cluster=w370, "library map"=w368, "start time"=w366) -> (w369:T8)
        n133 = call "Add State(s) to Queue__jki_lib_state_machine.vi"("State(s) in (\"\")"=w381) -> ("States Out"=w380:string)  [unwired: 14 in]
      }
      frame "Action: Listen for Client" {
        w395 = 100  # timeout
        # "Listen for Client.\n(Use this frame as the main \"throttle\" for timing)"
        n134 = Unbundle By Name(w398) -> ("listener ref"=w403:refnum<k5>)
        n135 = TCP Wait On Listener(8:w402, 9:w395, 11:w403) -> (0:w401:errorcluster, 4:w399:refnum<k5>)  [unwired: 4 out]
        n136 = case shown="No Error" w401 {
          selector: w401 -> [w411 w415]
          tunnel: [w411 w413] -> w400
          tunnel: w399 -> [w409 _]
          tunnel: w398 -> [w410 w412]
          tunnel: [w408 w412] -> w397
          tunnel: ["Action: Get Client Request" _] -> w396
          frame No Error {
            n137 = Bundle By Name(cluster=w410, "client ref"=w409) -> (w408:T8)
          }
          frame Error {
            # "No need to requeue listening state.  The timeout event will retrigger this state"
            # "Clear Timeout error.  Pass others"
            n138 = call <vilib>:"Clear Errors.vi"("error in (no error)"=w415, "specific error code to clear (0: all)"=56) -> ("error out"=w413:errorcluster)  [unwired: 4 in, 1 out]
          }
        }
        n139 = call "Add State(s) to Queue__jki_lib_state_machine.vi"("State(s) in Front (\"\")"=w396, "State(s) in (\"\")"=w406) -> ("States Out"=w405:string)  [unwired: 13 in]
      }
      frame "Action: Close TCP Port" {
        # "Listen for Client.\n(Use this frame as the main \"throttle\" for timing)"
        n140 = Unbundle By Name(w419) -> ("listener ref"=w418:refnum<k5>)
        n141 = TCP Close Connection(connection ID=w418, error in (no error)=w417) -> (error out=w416:errorcluster)  [unwired: 1 in, 1 out]
        n142 = call "Add State(s) to Queue__jki_lib_state_machine.vi"("State(s) in (\"\")"=w422) -> ("States Out"=w421:string)  [unwired: 14 in]
      }
      frame "Action: Open Listener" {
        w428 = 0  # timeout
        w429 = u16 6340  # port
        # "Clear error 56: timeout"
        # "Open TCP Port.\n(Open listener TCP port)"
        n143 = call <vilib>:"TCP Listen.vi"("error in (no error)"=w430, "timeout ms (wait forever: -1)"=w428, "port"=w429) -> ("error out"=w425:errorcluster, "listener ID"=w427:refnum<k5>)  [unwired: 4 in, 3 out]
        n144 = call <vilib>:"Clear Errors.vi"("error in (no error)"=w425, "specific error code to clear (0: all)"=56) -> ("error out"=w423:errorcluster)  [unwired: 4 in, 1 out]
        n145 = Bundle By Name(cluster=w431, "listener ref"=w427) -> (w426:T8)
        n146 = call "Add State(s) to Queue__jki_lib_state_machine.vi"("State(s) in (\"\")"=w434) -> ("States Out"=w433:string)  [unwired: 14 in]
      }
    }
  }
